vi "Get Foreign Key.vi"(8 "error in (no error)":errorcluster, 11 "Basic Column Configuration in":refnum<class "Basic Column Configuration.lvclass">) -> (0 "error out":errorcluster, 2 "FK Info":T1, 3 "Basic Column Configuration out":refnum<class "Basic Column Configuration.lvclass">)   [LabVIEW 2020, in "Basic Columns.lvlib" / "Basic Column Configuration.lvclass"]
uses:
  Basic Column Configuration.lvclass
  Legacy/Field/FK Info.ctl
  Basic Column Configuration.lvclass/Basic Column Configuration.ctl
  Column Interfaces.lvlib
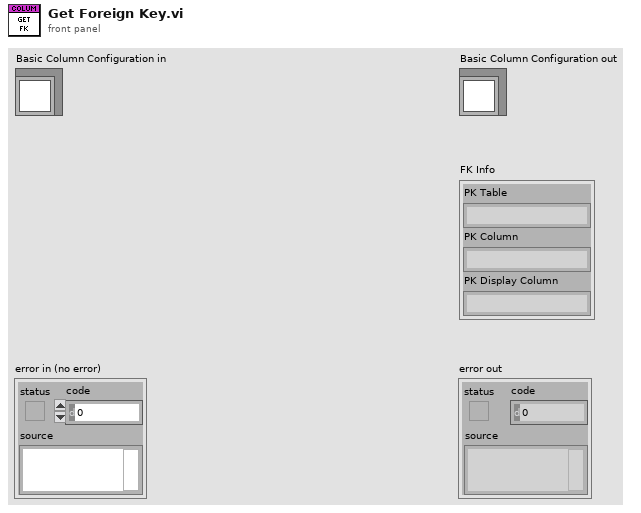
[diagram p1: front panel]
types:
  T1 = typedef "Column Interfaces.lvlib/FK Info.ctl" = cluster{"PK Table":string, "PK Column":string, "PK Display Column":string}
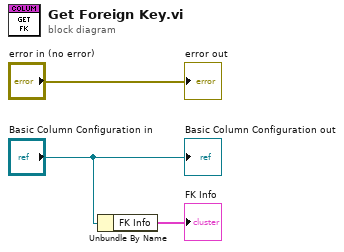
[diagram p0: block diagram]
diagram:
  n1 = Unbundle By Name("Basic Column Configuration in") -> ("FK Info"=→"FK Info":T1)
  "error out" <- "error in (no error)"
  "Basic Column Configuration out" <- "Basic Column Configuration in"
